vi "XMASSdll.vi"(8 "error in (no error)":errorcluster, 11 "xmol":dbl[](array[numeric])) -> (0 "error out":errorcluster, 2 "wmix out":dbl, 3 "xkg out":dbl[](array[numeric]))   [LabVIEW 2016]
doc: "subroutine XMASS (xmol,xkg,wmix)\n\nConverts composition on a mole fraction basis to mass fraction\n\nINPUTS:\n xmol--composition array [array of mol frac]\n\nOUTPUTS:\n xkg--composition array [array of mass frac]\n wmix--molar mass of the mixture [g/mol], a.k.a. \"molecular weight\""
uses:
  REFPROP.DLL
panel:
  # "REFPROP-XMASSdll.vi"
  # "void  XMASSdll(double *xmol, double *xkg, double *wmix)"
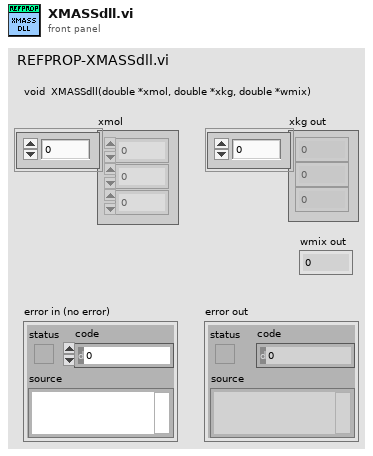
[diagram p1: front panel]
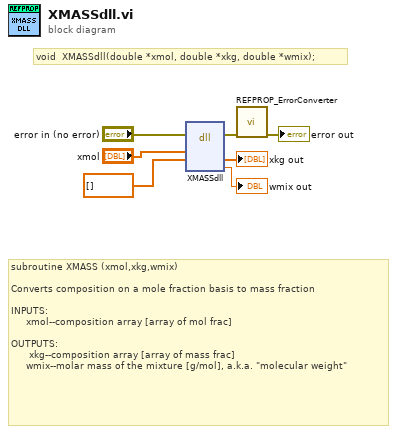
[diagram p0: block diagram]
diagram:
  # "void  XMASSdll(double *xmol, double *xkg, double *wmix);"
  # "subroutine XMASS (xmol,xkg,wmix)\n\nConverts composition on a mole fraction basis to mass fraction\n\nINPUTS:\n     xmol--composition array [array of mol frac]\n\nOUTPUTS:\n      xkg--composition array [array of mass frac]\n     wmix--molar mass of the mixture [g/mol], a.k.a. \"molecular weight\""
  n1 = dll-call lib="S:/009 - Testing/02 - Performance Testing/REFPROP/REFPROP.*" fn="XMASSdll"(error in="error in (no error)", "xmol"="xmol", "xkg"=dbl[] []) -> (error out=w4:errorcluster, "xkg"=→"xkg out":dbl[], "wmix"=→"wmix out":dbl)  [unwired: 5 in, 1 out]
  n2 = call "REFPROP_ErrorConverter.vi"("error in (no error)"=w4) -> ("error out"=→"error out":errorcluster)  [unwired: 10 in]
